vi "Add Copyright.vi"(8 "error in (no error)":errorcluster, 9 "Copyright Text":string, 10 "VI Index":i32, 11 "VI Data":T1[](array[typedef])) -> (0 "error out":errorcluster, 1 "VI Description":string, 3 "VI Data out":T1[](array[typedef]))   [LabVIEW 2023, in "VI Properties Editor.lvlib"]
uses:
  VI Properties Editor.lvlib
  Cluster Data.ctl
  <vilib>/picture/picture.llb/imagedata.ctl
  <vilib>/Utility/error.llb/Trim Whitespace One-Sided.vi
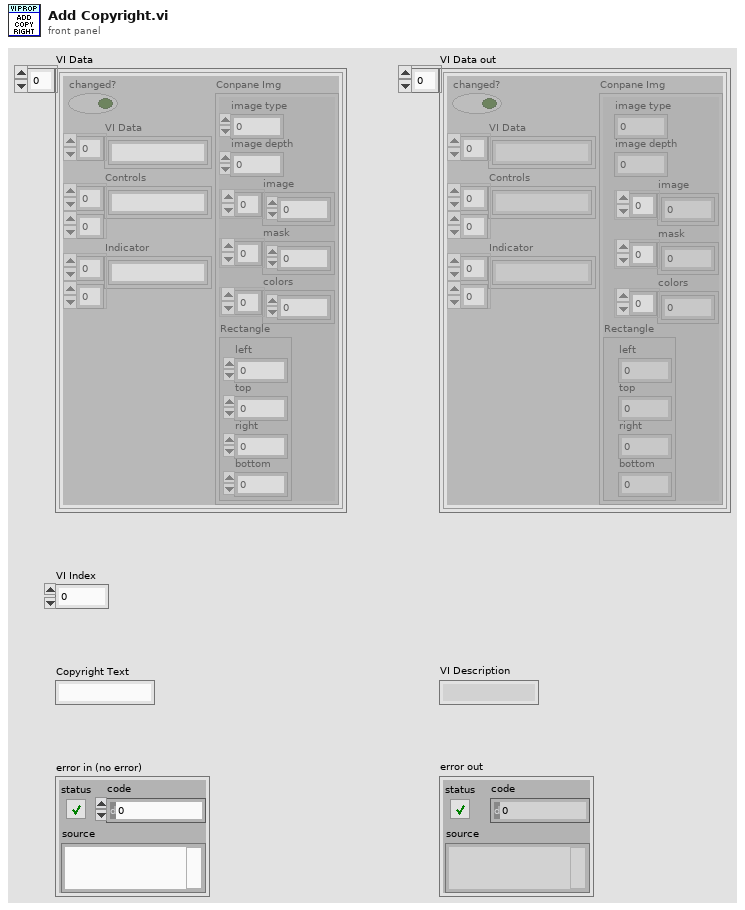
[diagram p1: front panel]
types:
  T1 = typedef "VI Properties Editor.lvlib/Cluster Data.ctl" = cluster{"changed?":bool, "VI Data":string[], "Controls":string[][], "Indicator":string[][], "Conpane Img":T2}
  T2 = typedef "imagedata.ctl" = cluster{"image type":i32, "image depth":i32, "image":u8[], "mask":u8[], "colors":u32[], "Rectangle":cluster{"left":i16, "top":i16, "right":i16, "bottom":i16}}
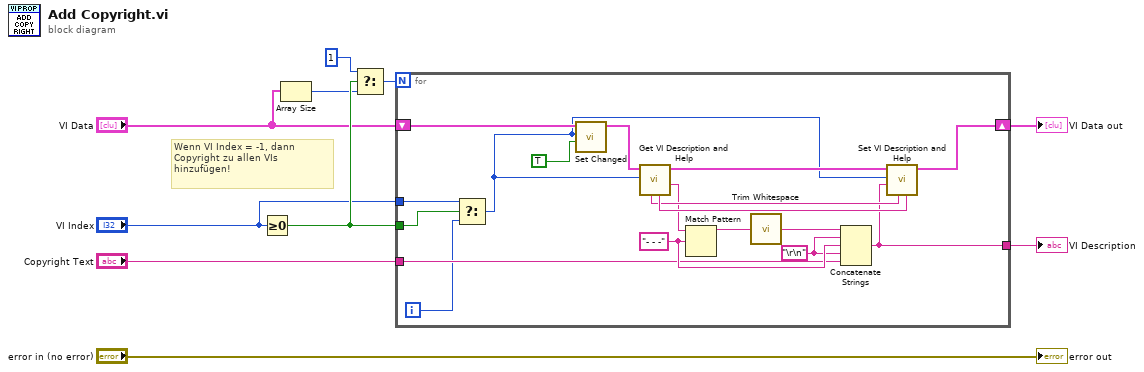
[diagram p0: block diagram]
diagram:
  # "Wenn VI Index = -1, dann Copyright zu allen VIs hinzufügen!"
  n1 = Greater Or Equal To 0?(x="VI Index") -> (x >= 0?=w10:bool)
  n2 = Array Size(array="VI Data") -> (size(s)=w7:i32)
  n3 = Select(t=1, s=w10, f=w7) -> (s? t:f=w9:i32)
  n4 = for {
    N: w9 -> [_]
    tunnel: "VI Index" -> [w14]
    tunnel: "Copyright Text" -> [w17]
    shift-right: [w22] -> w5
    shift-left: "VI Data" -> [w27]
    tunnel: w10 -> [w12]
    tunnel: [w11] -> w6
    i -> [w15]
    w18 = "\r\n"
    w19 = "- - -"
    n5 = Select(t=w14, s=w12, f=w15) -> (s? t:f=w13:i32)
    n6 = call "Set Changed.vi"("Changed?"=TRUE ("new element/subarray"), "VI Index"=w13, "VI Data in"=w27) -> ("VI Data out"=w26:T1[])  [unwired: 8 in]
    n7 = call "Get VI Description and Help.vi"("VI Index"=w13, "VI Data in"=w26) -> ("VI Description"=w21:string, "VI Data out"=w25:T1[], "Help Tag"=w24:string, "Help Path"=w23:string)  [unwired: 6 in]
    n8 = Match Pattern(string=w21, regular expression=w19) -> (before substring=w20:string)  [unwired: 1 in, 3 out]
    n9 = call <vilib>:"Trim Whitespace.vi"("string"=w20) -> ("trimmed string"=w16:string)  [unwired: 1 in]
    n10 = Concatenate Strings(w16, w18, w19, w18, w17) -> (w11:string)
    n11 = call "Set VI Description and Help.vi"("Help Tag"=w24, "Help Path"=w23, "VI Description"=w11, "VI Index"=w13, "VI Data in"=w25) -> ("VI Data out"=w22:T1[])  [unwired: 6 in]
  }
  "VI Data out" <- w5
  "VI Description" <- w6
  "error out" <- "error in (no error)"
